vi "SSL Detection Frame Balls Kalman Estimator.vi"(5 "Time Stamp 2":timestamp=timestamp(3583818425.330139 s since 1904-01-01), 7 "Life Time 2":dbl=0.2, 8 "ignora esquerda?":bool=TRUE, 9 "ignora lado":bool=TRUE, 11 "Detection Ball \nArray":T1[](array[typedef])) -> (3 "balls":T1[](array[typedef]))   [LabVIEW 2017]
uses:
  SSL Detection Ball.ctl
  <vilib>/Analysis/Matrix/Datatypes/RealMatrix.ctl
  <vilib>/Analysis/_algsub.llb/Real Vector Norm.vi
  <vilib>/Analysis/coordinate.llb/Wrap Angle (scalar).vi
  <vilib>/Analysis/Matrix/Numeric/Subtract/Subtract - RM,RM.vi
  <vilib>/Analysis/Matrix/NI_Matrix.lvlib
  <vilib>/Analysis/NI_AALPro.lvlib
  <vilib>/Analysis/NI_AAL_Angle.lvlib
panel:
  in  "Life Time":dbl=1.0
  in  "Array":T3(array[cluster])
  out "A - B":dbl[][](array[numeric])
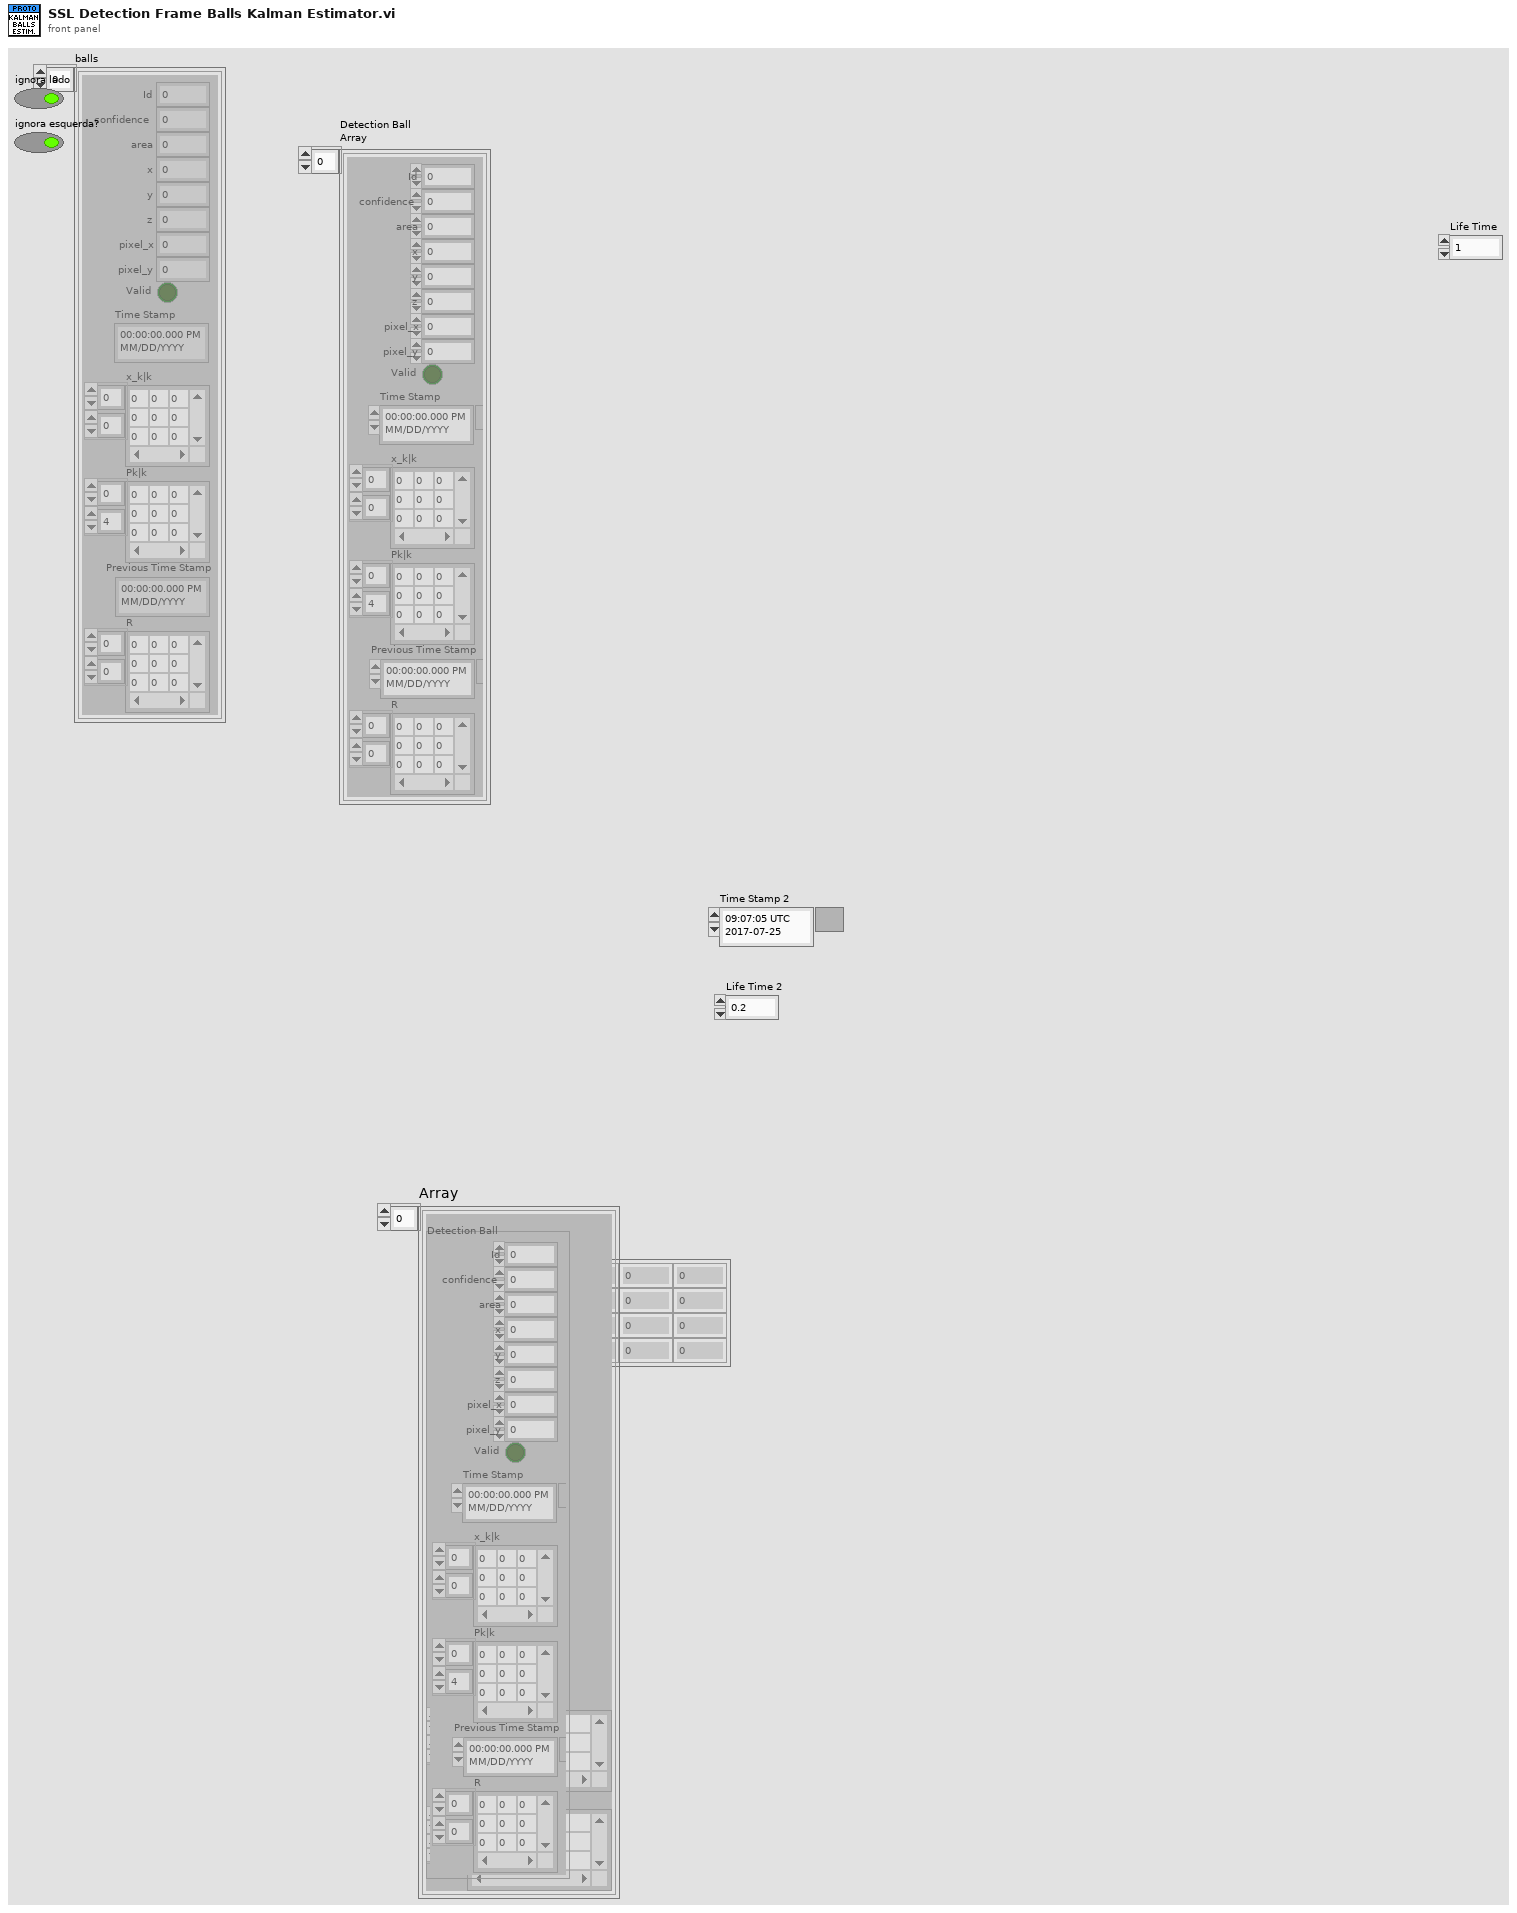
[diagram p1: front panel]
types:
  T1 = typedef "SSL Detection Ball.ctl" = cluster{"x":sgl, "area":u32, "confidence":sgl, "y":sgl, "z":sgl, "pixel_x":sgl, "pixel_y":sgl, "Valid":bool, "Time Stamp":timestamp, "x_k|k":T2, "Pk|k":T2, "Id":u32, "Previous Time Stamp":timestamp, "R":T2}
  T2 = typedef "NI_Matrix.lvlib/RealMatrix.ctl" = dbl[][]
  T3 = cluster{"Detection Ball":T1, "Pose":T2, "Pk|k":T2}[]
  T4 = cluster{"Detection Ball":T1, "Pose":T2, "Pk|k":T2}
  T5 = cluster{"Detection Ball out":T1, "x_k|k":T2, "Pk|k":T2}
  T6 = typedef "SSL Detection Ball.ctl" = cluster{"x":sgl, "area":u32, "confidence":sgl, "y":sgl, "z":sgl, "pixel_x":sgl, "pixel_y":sgl, "Valid":bool, "Time Stamp":timestamp, "x_k|k":T2, "Pk|k":T2, "ID#":dbl}
  T7 = cluster{"Detection Ball out":T1, "x_k|k":T2, "Pk|k":T2}[]
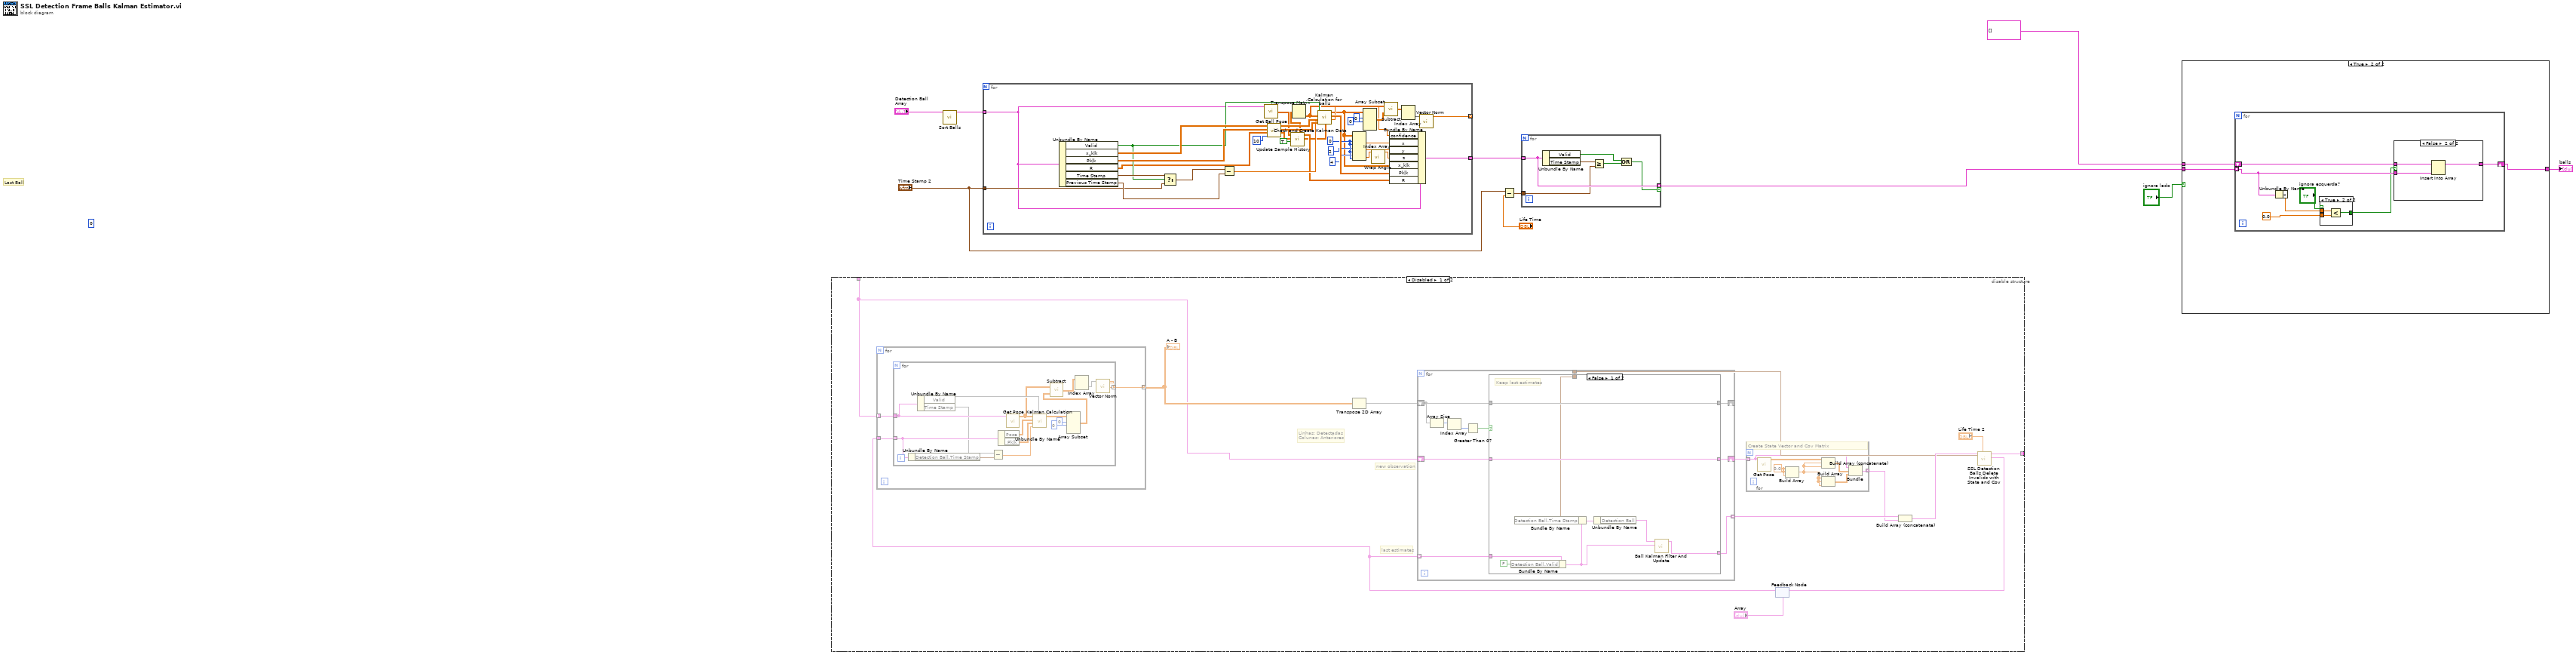
[diagram p0: block diagram]
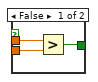
[diagram p3: hidden frame]
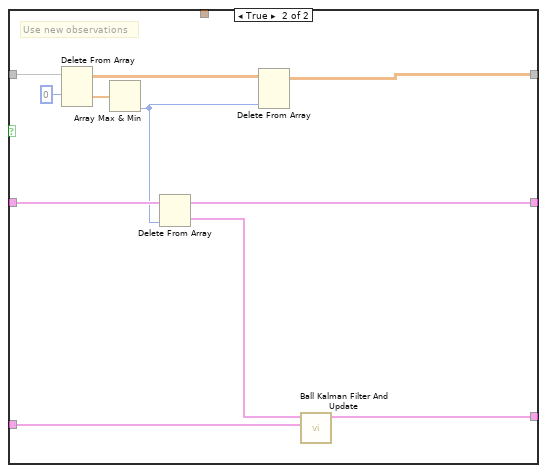
[diagram p5: hidden frame]
diagram:
  (unwired) u32 0 ("ID#")
  # "Last Ball"
  n1 = disable-structure shown="Disabled" {
    disable-tunnel: _ -> [w20 _]
    disable-tunnel: [w12 _] -> _
    frame Disabled {
      # "last estimates"
      # "new observation"
      # "Linhas: Detectadas\nColunas: Anteriores"
      n2 = feedback #1("Array") -> (w14:T3)
      n3 = for {
        tunnel: w14 -> [w63]
        tunnel: w20 -> [w62] mode=indexing
        tunnel: [w61] -> w22 mode=indexing
        n4 = for {
          tunnel: w63 -> [w67] mode=indexing
          tunnel: w62 -> [w79]
          tunnel: [w72] -> w61 mode=indexing
          n5 = Unbundle By Name(w67) -> ("Detection Ball.Time Stamp"=w66:timestamp)
          n6 = Unbundle By Name(w79) -> ("Valid"=w78, "Time Stamp"=w65)
          n7 = Subtract(x=w65, y=w66) -> (x-y=w64:dbl)
          n8 = Unbundle By Name(w67) -> ("Pose"=w69:T2, "Pk|k"=w68:T2)
          n9 = call-poly "Get Pose.vi"("Detection Ball"=w79) -> ("Pose"=w77:T2)  [unwired: 10 in]
          n10 = call "Kalman Calculation.vi"("Use Observation"=w78, "intervalo"=w64, "Pk-1|k-1"=w68, "x_k-1|k-1"=w69, "z_k"=w77) -> ("x_k|k"=w75:T2)  [unwired: 4 in, 2 out]
          n11 = Array Subset(array=w75, index (row)=0 ("row 1"), length (row)=0 ("row N")) -> (w76:T2)  [unwired: 2 in]
          n12 = call-poly <vilib>:"Subtract.vi"("Real Matrix B"=w76, "Real Matrix A"=w77) -> ("A - B"=w71:T2)
          n13 = Index Array(array=w71) -> (element=w70:dbl[])  [unwired: 2 in]
          n14 = call-poly <vilib>:"Vector Norm.vi"("Input Vector"=w70) -> ("norm"=w72:dbl)  [unwired: 9 in, 1 out]
        }
      }
      "A - B" <- w22
      n15 = Transpose 2D Array(2D array=w22) -> (transposed array=w23:dbl[][])
      n16 = for {
        shift-right: [w39] -> _
        shift-left: w23 -> [w35]
        shift-right: [w38] -> w21
        shift-left: w20 -> [w40]
        tunnel: [w37] -> w19 mode=indexing
        tunnel: w14 -> [w36] mode=indexing
        tunnel: w13 -> [w31]
        n17 = Array Size(array=w35) -> (size(s)=w33:i32[])
        n18 = Index Array(array=w33) -> (element=w32:i32)  [unwired: 1 in]
        n19 = Greater Than 0?(x=w32) -> (x > 0?=w34:bool)
        n20 = case shown="False" w34 {
          tunnel: w35 -> [w49 w60]
          tunnel: w40 -> [w48 w57]
          tunnel: [w49 w55] -> w39
          tunnel: [w48 w53] -> w38
          tunnel: [w41 w52] -> w37
          tunnel: w36 -> [w46 w50]
          tunnel: w31 -> [w44 _]
          frame False {
            # "Keep last estimates"
            n21 = Bundle By Name(cluster=w46, "Detection Ball.Valid"=FALSE) -> (w45:T4)
            n22 = Bundle By Name(cluster=w45, "Detection Ball.Time Stamp"=w44) -> (w43:T4)
            n23 = Unbundle By Name(w43) -> ("Detection Ball"=w42:T1)
            n24 = call "Ball Kalman Filter And Update.vi"("Cluster in"=w45, "Detection Ball"=w42) -> ("Cluster out"=w41:T5)  [unwired: 9 in]
          }
          frame True {
            # "Use new observations"
            n25 = Delete From Array(array=w60, index (row)=0) -> (deleted portion=w58:dbl[], array with subset deleted=w56:dbl[][])  [unwired: 2 in]
            n26 = Array Max & Min(array=w58) -> (min index (indices)=w54:i32)  [unwired: 3 out]
            n27 = Delete From Array(array=w57, index=w54) -> (deleted portion=w51:T6, array with subset deleted=w53:T6[])  [unwired: 1 in]
            n28 = Delete From Array(array=w56, index (col)=w54) -> (array with subset deleted=w55:dbl[][])  [unwired: 2 in, 1 out]
            n29 = call "Ball Kalman Filter And Update.vi"("Cluster in"=w50, "Detection Ball"=w51) -> ("Cluster out"=w52:T5)  [unwired: 9 in]
          }
        }
      }
      n30 = for {
        tunnel: w21 -> [w24] mode=indexing
        tunnel: [w25] -> w18 mode=indexing
        w30 = 0.0 ("element")
        # "Create State Vector and Cov Matrix"
        n31 = call-poly "Get Pose.vi"("Detection Ball"=w24) -> ("Pose"=w28:T2)  [unwired: 10 in]
        n32 = Build Array(w30, w30, w30) -> (w29:dbl[])
        n33 = Build Array(w29, w29, w29) -> (w27:dbl[][])
        n34 = Build Array (concatenate)(w28, w29, w29) -> (w26:T2)
        n35 = Bundle("Detection Ball"=w24, "Pose"=w26, w27) -> (w25:cluster{"Detection Ball":T6, "Pose":T2, dbl[][]})  [unwired: 1 in]
      }
      n36 = Build Array (concatenate)(w19, w18) -> (w16:T7)
      n37 = call "SSL Detection Balls Delete Invalids with State and Cov.vi"("Life Time"="Life Time 2", "Array"=w16) -> ("Array 2"=w11:T3, "Balls Out"=w12:T1[], "Now"=w13:timestamp)  [unwired: 7 in]
      n38 = feedback-in #1(w11) -> ()
    }
    frame Enabled {
    }
  }
  n39 = call "Sort Balls.vi"("Detection Ball \nArray"="Detection Ball \nArray") -> ("Sorted Detection Ball \nArray"=w4:T1[])  [unwired: 10 in]
  n40 = for {
    tunnel: w4 -> [w82] mode=indexing
    tunnel: [w116] -> _ mode=indexing
    tunnel: [w84] -> w6 mode=indexing
    tunnel: "Time Stamp 2" -> [w102]
    w97 = 0 ("index (row)")
    n41 = Unbundle By Name(w82) -> ("Valid"=w100:bool, "x_k|k"=w109:T2, "Pk|k"=w107:T2, "R"=w94:T2, "Time Stamp"=w103:timestamp, "Previous Time Stamp"=w105:timestamp)
    n42 = Select(t=w103, s=w100, f=w102) -> (s? t:f=w101:timestamp)
    n43 = Subtract(x=w101, y=w105) -> (x-y=w104:dbl)
    n44 = call "Get Ball Pose.vi"("Detection Ball"=w82) -> ("Pose"=w83:T2)  [unwired: 10 in]
    n45 = call "Check and Create Kalman Data.vi"("Variance Memory"=10, "R"=w94, "Pk"=w107, "x_k"=w109) -> ("R out"=w93:T2, "Pk out"=w106:T2, "x_k out"=w108:T2)  [unwired: 5 in]
    n46 = call "Update Sample History.vi"("Ball?"=TRUE, "R in"=w93, "Sample"=w83) -> ("covariance matrix V"=w89:T2, "R out"=w90:T2, "Sample Unwrapped"=w88:T2)  [unwired: 6 in]
    n47 = Transpose Matrix(1:w88) -> (0:w91:T2)
    n48 = call "Kalman Calculation for balls.vi"("R"=w89, "intervalo"=w104, "Pk-1|k-1"=w106, "x_k-1|k-1"=w108, "z_k"=w91, "Use Observation"=w100) -> ("Conf"=w85:dbl, "Pk|k"=w110:T2, "x_k|k"=w81:T2)  [unwired: 3 in]
    n49 = Index Array(array=w81, index (row) #1=w97, index (col) #1=w97, index (row) #2=2 ("disabled index (col)"), index (col) #2=w97, index (row) #3=4 ("disabled index (col)"), index (col) #3=w97) -> (element #1=w99:dbl, element #2=w98:dbl, element #3=w87:dbl)
    n50 = Array Subset(array=w81, index (row)=0 ("row 1"), length (row)=0 ("row N")) -> (w115:T2)  [unwired: 2 in]
    n51 = call-poly <vilib>:"Wrap Angle.vi"("angle in"=w87) -> ("angle out"=w86:dbl)  [unwired: 9 in, 1 out]
    n52 = call-poly <vilib>:"Subtract.vi"("Real Matrix B"=w115, "Real Matrix A"=w91) -> ("A - B"=w112:T2)
    n53 = Bundle By Name(cluster=w82, "confidence"=w85, "x"=w99, "y"=w98, "z"=w86, "x_k|k"=w81, "Pk|k"=w110, "R"=w90) -> (w84:T1)
    n54 = Index Array(array=w112) -> (element=w111:dbl[])  [unwired: 2 in]
    n55 = call-poly <vilib>:"Vector Norm.vi"("Input Vector"=w111) -> ("norm"=w116:dbl)  [unwired: 9 in, 1 out]
  }
  n56 = Subtract(x="Time Stamp 2", y="Life Time") -> (x-y=w7:timestamp)
  n57 = for {
    tunnel: w6 -> [w122] mode=indexing
    tunnel: [w122] -> w3 mode=indexing if=w121
    tunnel: w7 -> [w119]
    n58 = Unbundle By Name(w122) -> ("Valid"=w118:bool, "Time Stamp"=w120:timestamp)
    n59 = Greater Or Equal?(x=w120, y=w119) -> (x >= y?=w117:bool)
    n60 = Compound Arithmetic op=OR(w118, w117) -> (w121:bool)
  }
  n61 = case shown="True" "ignora lado" {
    tunnel: w3 -> [w123 w126]
    tunnel: T1[] [] -> [_ w125]
    tunnel: [w123 w124] -> w10
    frame False {
    }
    frame True {
      n62 = for {
        tunnel: w126 -> [w131] mode=indexing
        shift-right: [w133] -> w124
        shift-left: w125 -> [w132]
        n63 = Unbundle By Name(w131) -> ("x"=w130:sgl)
        n64 = case shown="True" "ignora esquerda?" {
          tunnel: w130 -> [w136 w139]
          tunnel: sgl 0.0 ("y") -> [w135 w138]
          tunnel: [w134 w137] -> w128
          frame False {
            n65 = Greater?(x=w136, y=w135) -> (0:w134:bool)
          }
          frame True {
            n66 = Less?(x=w139, y=w138) -> (x < y?=w137:bool)
          }
        }
        n67 = case shown="False" w128 {
          tunnel: w131 -> [_ w143]
          tunnel: [w140 w142] -> w133
          tunnel: w132 -> [w140 w141]
          frame True {
          }
          frame False {
            n68 = Insert Into Array(array=w141, new element=w143) -> (w142:T1[])  [unwired: 1 in]
          }
        }
      }
    }
  }
  "balls" <- w10
